vi "RTK last 10 nema returns.vi"(11 "x":string) -> (3 "Array":string[](array[string]))   [LabVIEW 2009]
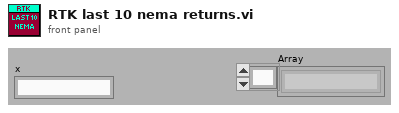
[diagram p1: front panel]
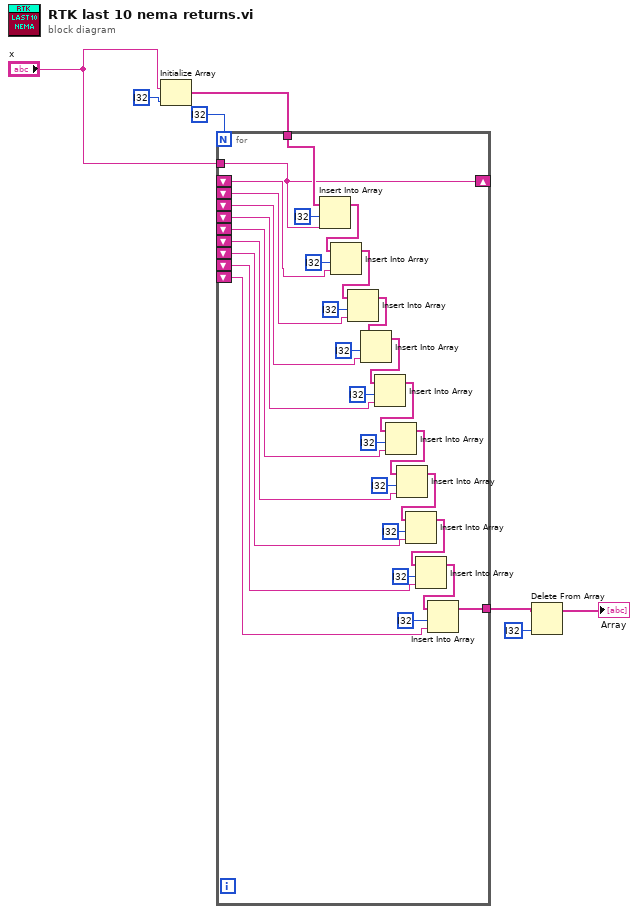
[diagram p0: block diagram]
diagram:
  n1 = Initialize Array("x", i32 ? ("dimension size")) -> (w6:string[])
  n2 = for {
    N: i32 ? -> [_]
    shift-right: [w8] -> _
    shift-left: _ -> [w18]
    shift-left: _ -> [w17]
    shift-left: _ -> [w16]
    shift-left: _ -> [w15]
    shift-left: _ -> [w14]
    shift-left: _ -> [w13]
    shift-left: _ -> [w12]
    shift-left: _ -> [w11]
    shift-left: _ -> [w10]
    tunnel: w6 -> [w38]
    tunnel: [w9] -> w3
    tunnel: "x" -> [w8]
    n3 = Insert Into Array(array=w38, index=i32 ?, new element=w8) -> (w36:string[])
    n4 = Insert Into Array(array=w36, index=i32 ?, new element=w18) -> (w35:string[])
    n5 = Insert Into Array(array=w35, index=i32 ?, new element=w17) -> (w34:string[])
    n6 = Insert Into Array(array=w34, index=i32 ?, new element=w16) -> (w33:string[])
    n7 = Insert Into Array(array=w33, index=i32 ?, new element=w15) -> (w32:string[])
    n8 = Insert Into Array(array=w32, index=i32 ?, new element=w14) -> (w31:string[])
    n9 = Insert Into Array(array=w31, index=i32 ?, new element=w13) -> (w30:string[])
    n10 = Insert Into Array(array=w30, index=i32 ?, new element=w12) -> (w29:string[])
    n11 = Insert Into Array(array=w29, index=i32 ?, new element=w11) -> (w28:string[])
    n12 = Insert Into Array(array=w28, index=i32 ?, new element=w10) -> (w9:string[])
  }
  n13 = Delete From Array(array=w3, index=i32 ?) -> (array with subset deleted=→"Array":string[])  [unwired: 1 in, 1 out]
